vi "IO.vi"(8 "错误常量":errorcluster, 9 "DO DATA":bool[](array[boolean]), 10 "IO Name":string[](array[string]), 11 "IO?":enum16{"DI", "DO"}(ring)=enum."DO") -> (0 "error out":errorcluster, 2 "IO Data":string[][](array[string]), 3 "DI":bool[](array[boolean]))   [LabVIEW 2017]
uses:
  Adlink IO/Adlink IO.lvlib
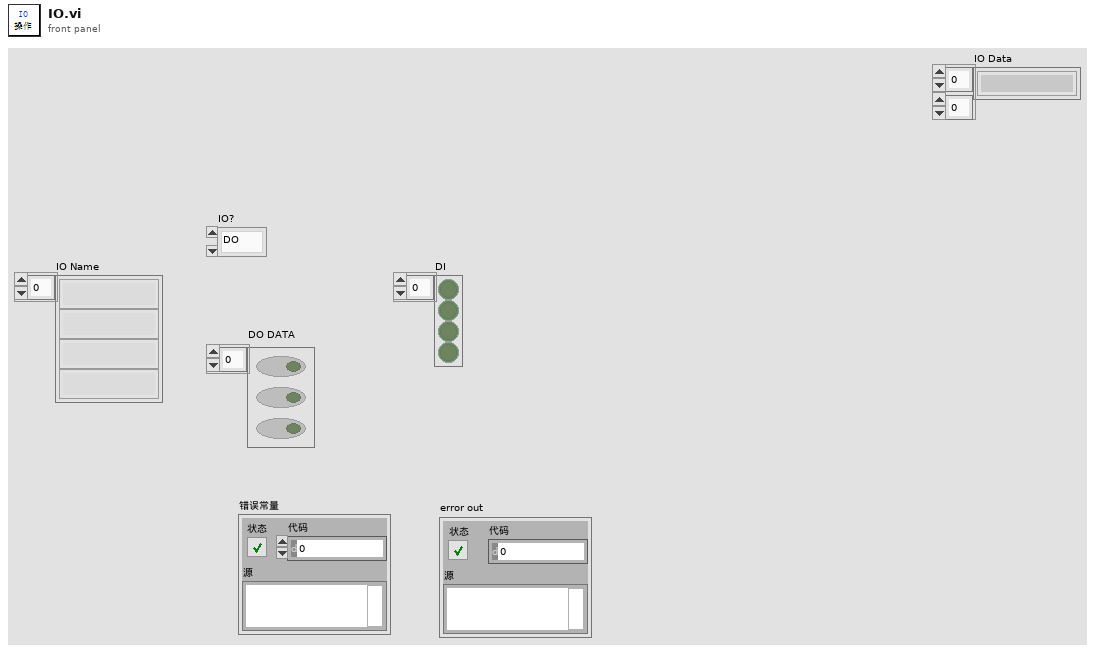
[diagram p1: front panel]
types:
  T1 = cluster{"DI dev":i32[], "DI line":i32[], "Port":i32[], "DO dev":i32[], "DO line":i32[], "IO Data":string[][], "IO f":i16[]}
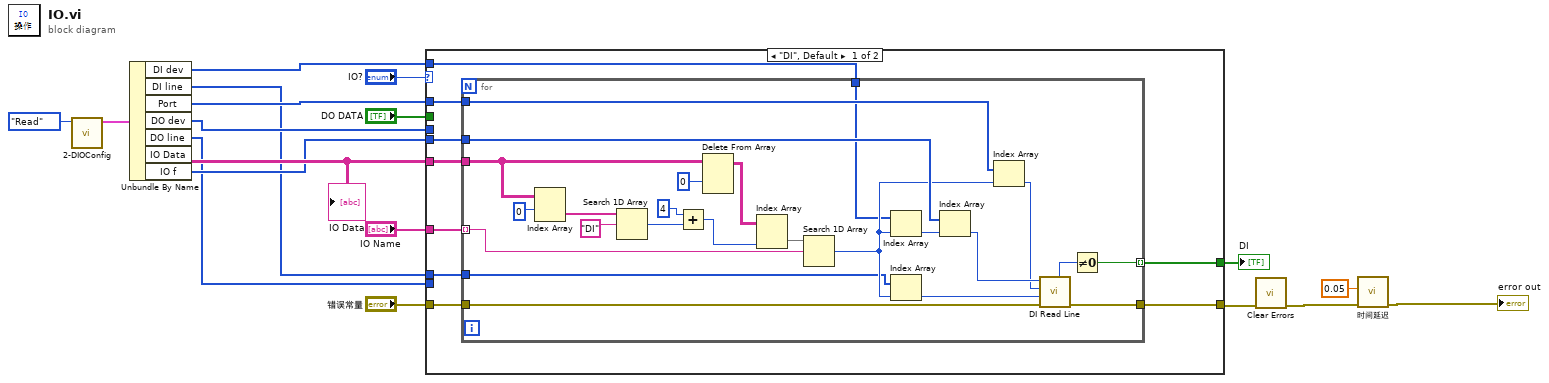
[diagram p0: block diagram]
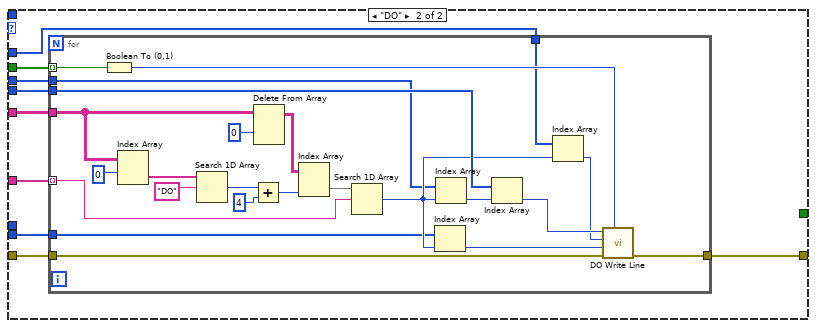
[diagram p2: hidden frame]
diagram:
  n1 = call "2-DIOConfig.vi"("Step"=enum16{"Initial", "Write", "Read"}."Read") -> ("DIO pra out"=w5:T1)  [unwired: 9 in, 1 out]
  n2 = Unbundle By Name(w5) -> ("DI dev"=w7:i32[], "DI line"=w6:i32[], "Port"=w8:i32[], "DO dev"=w10:i32[], "DO line"=w9:i32[], "IO Data"=w12:string[][], "IO f"=w11:i16[])
  "IO Data" <- w12
  n3 = case shown="\"DI\", Default" "IO?" {
    tunnel: w12 -> [w27 w59]
    tunnel: "IO Name" -> [w26 w60]
    tunnel: [w25 _] -> w17
    tunnel: "DO DATA" -> [_ w58]
    tunnel: "错误常量" -> [w24 w57]
    tunnel: [w23 w56] -> w13
    tunnel: w11 -> [w22 w55]
    tunnel: w10 -> [_ w54]
    tunnel: w9 -> [_ w53]
    tunnel: w8 -> [w21 w52]
    tunnel: w7 -> [w20 _]
    tunnel: w6 -> [w19 _]
    frame "DI", Default {
      n4 = for {
        tunnel: w27 -> [w38]
        tunnel: w26 -> [w44] mode=indexing
        tunnel: [w43] -> w25 mode=indexing
        tunnel: [w41] -> w23
        tunnel: w24 -> [w42]
        tunnel: w22 -> [w36]
        tunnel: w21 -> [w30]
        tunnel: w20 -> [w29]
        tunnel: w19 -> [w28]
        n5 = Index Array(array=w38, index (row)=0 ("索引 (行)")) -> (element=w50:string[])  [unwired: 1 in]
        n6 = Search 1D Array(1D array=w50, element="DI" ("元素")) -> (index of element=w45:i32)  [unwired: 1 in]
        n7 = Add(x=4 ("y"), y=w45) -> (x+y=w47:i32)
        n8 = Delete From Array(array=w38, index (row)=0 ("索引 (行)")) -> (array with subset deleted=w37:string[][])  [unwired: 2 in, 1 out]
        n9 = Index Array(array=w37, index (col)=w47) -> (element=w46:string[])  [unwired: 1 in]
        n10 = Search 1D Array(1D array=w46, element=w44) -> (index of element=w32:i32)  [unwired: 1 in]
        n11 = Index Array(array=w29, index=w32) -> (element=w33:i32)
        n12 = Index Array(array=w28, index=w32) -> (element=w40:i32)
        n13 = Index Array(array=w36, index=w33) -> (element=w35:i16)
        n14 = Index Array(array=w30, index=w32) -> (element=w31:i32)
        n15 = call "DI Read Line.vi"("error in (no error)"=w42, "Line"=w40, "Port"=w31, "CardNumber"=w35) -> ("error out"=w41:errorcluster, "State out"=w34:u16)  [unwired: 5 in, 1 out]
        n16 = Not Equal To 0?(x=w34) -> (x != 0?=w43:bool)
      }
    }
    frame "DO" {
      n17 = for {
        tunnel: w60 -> [w78] mode=indexing
        tunnel: w59 -> [w71]
        tunnel: w58 -> [w76] mode=indexing
        tunnel: w57 -> [w75]
        tunnel: [w74] -> w56
        tunnel: w55 -> [w68]
        tunnel: w54 -> [w63]
        tunnel: w53 -> [w62]
        tunnel: w52 -> [w61]
        n18 = Boolean To (0,1)(Boolean=w76) -> (0, 1=w67:i16)
        n19 = Index Array(array=w71, index (row)=0 ("索引 (行)")) -> (element=w83:string[])  [unwired: 1 in]
        n20 = Search 1D Array(1D array=w83, element="DO" ("元素")) -> (index of element=w77:i32)  [unwired: 1 in]
        n21 = Add(x=w77, y=4) -> (x+y=w80:i32)
        n22 = Delete From Array(array=w71, index (row)=0 ("索引 (行)")) -> (array with subset deleted=w69:string[][])  [unwired: 2 in, 1 out]
        n23 = Index Array(array=w69, index (col)=w80) -> (element=w79:string[])  [unwired: 1 in]
        n24 = Search 1D Array(1D array=w79, element=w78) -> (index of element=w65:i32)  [unwired: 1 in]
        n25 = Index Array(array=w62, index=w65) -> (element=w72:i32)
        n26 = Index Array(array=w63, index=w65) -> (element=w73:i32)
        n27 = Index Array(array=w68, index=w73) -> (element=w66:i16)
        n28 = Index Array(array=w61, index=w65) -> (element=w64:i32)
        n29 = call "DO Write Line.vi"("Value"=w67, "error in (no error)"=w75, "Line"=w72, "Port"=w64, "CardNumber"=w66) -> ("error out"=w74:errorcluster)  [unwired: 5 in, 1 out]
      }
    }
  }
  "DI" <- w17
  n30 = call <vilib>:"Clear Errors.vi"("error in (no error)"=w13) -> ("error out"=w2:errorcluster)  [unwired: 5 in, 1 out]
  n31 = call "时间延迟"("error in (no error)"=w2, "Delay Time (s)"=0.05) -> ("error out"=→"error out":errorcluster)  [unwired: 9 in]
